vi "S2C_ExeScriptError.vi"(8 "Error In":errorcluster, 11 "Q-Ref":refnum<queue>) -> (0 "Error Out":errorcluster)   [LabVIEW 2015]
doc: "Changes the testing status to Error and calls the results case."
uses:
  Controls/S2C_ResultStatus.ctl
  Controls/S2C_ExePause.ctl
  Globals/S2C_Globals.vi
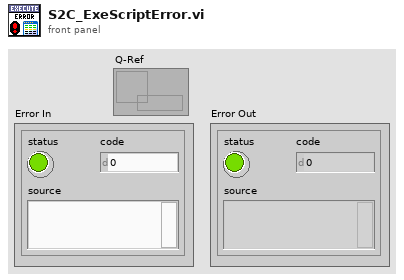
[diagram p1: front panel]
types:
  T1 = typedef "S2C_ExePause.ctl" = bool
  T2 = typedef "S2C_ResultStatus.ctl" = enum16{"Passed", "Failed", "Logged", "Aborted", "Error", "Testing...", "Paused", "No Record"}
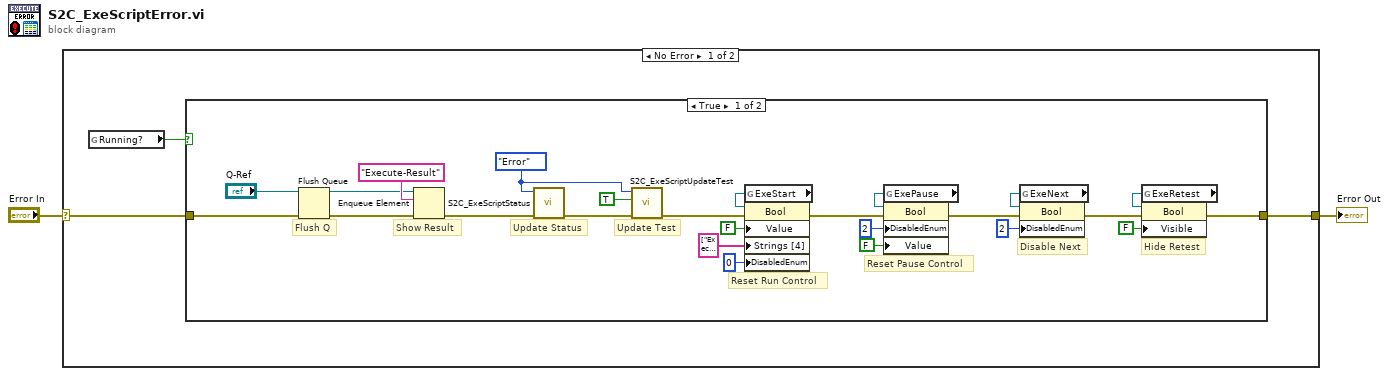
[diagram p0: block diagram]
diagram:
  n1 = case shown="No Error" "Error In" {
    selector: "Error In" -> [w3 w32]
    tunnel: [w4 w32] -> w1
    frame No Error {
      n2 = global read "S2C_Globals.vi" "Running?"() -> (w5:bool)
      n3 = case shown="True" w5 {
        tunnel: [w7 w31] -> w4
        tunnel: w3 -> [w14 w31]
        frame True {
          w15 = S2C_ResultStatus."Error" ("Status")
          # "Hide Retest"
          # "Flush Q"
          # "Update Test"
          # "Show Result"
          # "Reset Pause Control"
          # "Disable Next"
          # "Update Status"
          # "Reset Run Control"
          n4 = Flush Queue(queue="Q-Ref", error in (no error)=w14) -> (queue out=w11:refnum<queue>, error out=w13:errorcluster)  [unwired: 1 out]
          n5 = Enqueue Element(queue=w11, element="Execute-Result", error in (no error)=w13) -> (error out=w18:errorcluster)  [unwired: 1 in, 2 out]
          n6 = call "S2C_ExeScriptStatus.vi"("Error In"=w18, "Status"=w15) -> ("Error Out"=w17:errorcluster)  [unwired: 9 in]
          n7 = call "S2C_ExeScriptUpdateTest.vi"("Error In"=w17, "LastMeas?"=TRUE, "Status"=w15) -> ("Error Out"=w16:errorcluster)  [unwired: 8 in]
          n8 = global read "S2C_Globals.vi" "ExeStart"() -> (w29:refnum<vi>)
          n9 = property on="Property Node" class="Bool"(reference=w29, error in=w16, "Value"=FALSE ("Run"), "Strings [4]"=string[] ["Execute Script", "Abort Testing"] ("Array - String"), "DisabledEnum"=u8 0) -> (error out=w22:errorcluster)  [unwired: 1 out]
          n10 = global read "S2C_Globals.vi" "ExePause"() -> (w25:refnum<vi>)
          n11 = property on="Property Node" class="Bool"(reference=w25, error in=w22, "DisabledEnum"=u8 2, "Value"=T1 FALSE) -> (error out=w23:errorcluster)  [unwired: 1 out]
          n12 = global read "S2C_Globals.vi" "ExeNext"() -> (w28:refnum<vi>)
          n13 = property on="Property Node" class="Bool"(reference=w28, error in=w23, "DisabledEnum"=u8 2) -> (error out=w9:errorcluster)  [unwired: 1 out]
          n14 = global read "S2C_Globals.vi" "ExeRetest"() -> (w10:refnum<vi>)
          n15 = property on="Property Node" class="Bool"(reference=w10, error in=w9, "Visible"=FALSE) -> (error out=w7:errorcluster)  [unwired: 1 out]
        }
        frame False {
          # "Currently not running"
        }
      }
    }
    frame Error {
    }
  }
  "Error Out" <- w1
